vi "Find Packed Libraries.vi"(8 "error in (no error)":errorcluster, 11 "Transceiver Loader in":refnum<class "Transceiver Loader.lvclass">) -> (0 "error out":errorcluster, 2 "packed library paths":path[](array[path]), 3 "Transceiver Loader out":refnum<class "Transceiver Loader.lvclass">)   [LabVIEW 2017, in "Data Sharing Framework Core.lvlib" / "Data Sharing Framework Engine.lvlib" / "Transceiver Loader.lvclass"]
uses:
  Transceiver Loader.lvclass
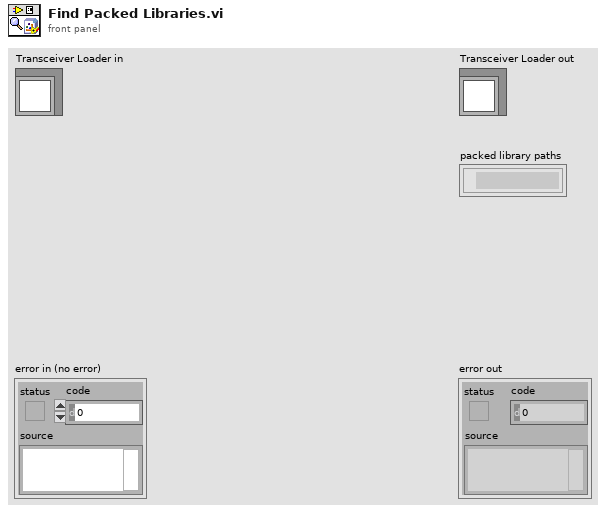
[diagram p1: front panel]
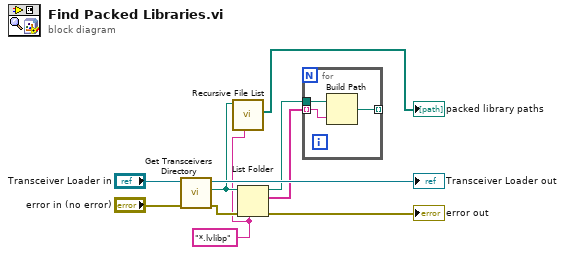
[diagram p0: block diagram]
diagram:
  w2 = "*.lvlibp" ("pattern")
  n1 = call "Get Transceivers Directory.vi"("error in (no error)"="error in (no error)", "Transceiver Loader in"="Transceiver Loader in") -> ("error out"=w6:errorcluster, "transceivers directory"=w3:path, "Transceiver Loader out"=→"Transceiver Loader out":refnum<class "Transceiver Loader.lvclass">)  [unwired: 7 in]
  n2 = call <vilib>:"Recursive File List.vi"("pattern"=w2, "Folder Path"=w3) -> ("All Files in Dir"=→"packed library paths":path[])  [unwired: 5 in, 4 out]
  n3 = List Folder(path=w3, pattern=w2, error in=w6) -> (path out=w7:path, filenames=w5:string[], error out=→"error out":errorcluster)  [unwired: 1 in, 1 out]
  n4 = for {
    tunnel: w5 -> [w12] mode=indexing
    tunnel: w7 -> [w13]
    tunnel: [w11] -> _ mode=indexing
    n5 = Build Path(base path=w13, name or relative path=w12) -> (appended path=w11:path)
  }
